vi "Read Modules.vi"(8 "error in (no error)":errorcluster, 11 "IO Loop in":refnum<class "Module Loop.lvclass">) -> (0 "error out":errorcluster, 2 "Modules":refnum<class "Module.lvclass">[](array[class]), 3 "IO Loop out":refnum<class "Module Loop.lvclass">)   [LabVIEW 2015, in "Module Loop.lvclass"]
uses:
  Module Loop.lvclass
  Module/Module/Module.lvclass
  Module Loop.lvclass/Module Loop.ctl
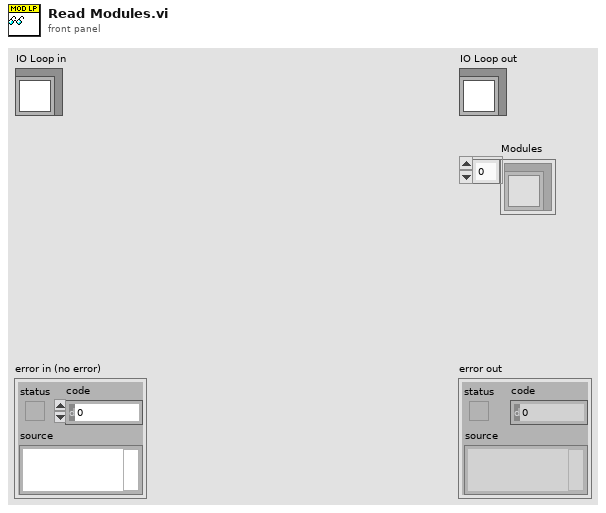
[diagram p1: front panel]
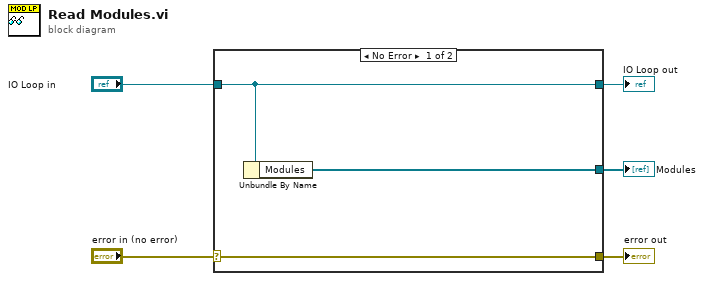
[diagram p0: block diagram]
diagram:
  n1 = case shown="No Error" "error in (no error)" {
    selector: "error in (no error)" -> [w8 w9]
    tunnel: [w8 w9] -> w4
    tunnel: [w7 w10] -> w2
    tunnel: "IO Loop in" -> [w7 w10]
    tunnel: [w6 _] -> w1
    frame No Error {
      n2 = Unbundle By Name(w7) -> ("Modules"=w6:refnum<class "Module.lvclass">[])
    }
    frame Error {
    }
  }
  "error out" <- w4
  "IO Loop out" <- w2
  "Modules" <- w1
